vi "Shed.vi"(8 "error in (no error)":errorcluster, 11 "SCADA in":refnum<class "SCADA.lvclass">) -> (0 "error out":errorcluster, 3 "SCADA out":refnum<class "SCADA.lvclass">)   [LabVIEW 2015, in "SCADA Core.lvlib" / "SCADA.lvclass"]
uses:
  SCADA.lvclass
  SCADA.lvclass/SCADA.ctl
  Controls/Queue Selector.ctl
  <vilib>/ActorFramework/Message Enqueuer/Message Enqueuer.lvclass/Message Enqueuer.ctl
  <vilib>/ActorFramework/Message Enqueuer/Enqueue.vi
  <vilib>/ActorFramework/Message Priority Queue/Priority Enqueue.vi
  IED Actor/IED Messages/Emergency Device Deactivate Msg/Emergency Device Deactivate Msg.lvclass
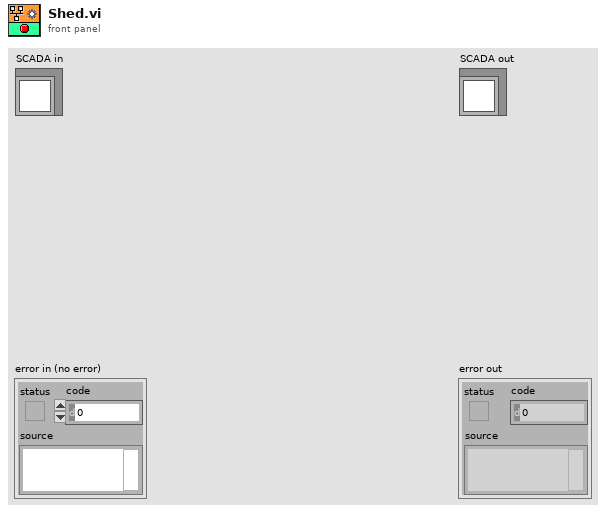
[diagram p1: front panel]
types:
  T1 = typedef "SCADA Core.lvlib/SCADA.lvclass/Queue Selector.ctl" = enum16{"IEDs", "PV", "Generators", "Wind", "Storage", "Relays"}
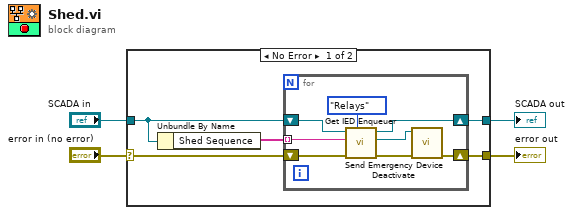
[diagram p0: block diagram]
diagram:
  n1 = case shown="No Error" "error in (no error)" {
    selector: "error in (no error)" -> [w8 w19]
    tunnel: [w5 w19] -> w3
    tunnel: [w6 w18] -> w1
    tunnel: "SCADA in" -> [w7 w18]
    frame No Error {
      n2 = Unbundle By Name(w7) -> ("Shed Sequence"=w9:string[])
      n3 = for {
        tunnel: w9 -> [w17] mode=indexing
        shift-right: [w10] -> w5
        shift-left: w8 -> [w16]
        shift-right: [w13] -> w6
        shift-left: w7 -> [w14]
        n4 = call "Get IED Enqueuer.vi"("Queue (IEDs)"=Queue_Selector."Relays" ("Queue"), "error in (no error)"=w16, "IED Name"=w17, "SCADA in"=w14) -> ("error out"=w11:errorcluster, "IED Enqueuer"=w12:refnum<class "Message Enqueuer.lvclass">, "SCADA out"=w13:refnum<class "SCADA.lvclass">)  [unwired: 5 in]
        n5 = call "Send Emergency Device Deactivate.vi"("error in (no error)"=w11, "Message Enqueuer"=w12) -> ("error out"=w10:errorcluster)  [unwired: 8 in, 1 out]
      }
    }
    frame Error {
    }
  }
  "error out" <- w3
  "SCADA out" <- w1
